vi "Verify File.vi"(5 "Options":T1, 7 "Test VI (caller)":string, 8 "error in":errorcluster, 9 "Extension":string, 10 "Path to Binary File to Verify":path) -> (0 "error out":errorcluster, 1 "Failure Message":string, 2 "Passed?":bool)   [LabVIEW 2020, in "Approval Tests.lvlib"]
doc: "Performs an approval test.\n\nThe first call, the test passes and the test data is written to the approved file.\n\nOn subsequent runs the test data is compared to the contents of the approved file.\nIf it is a match, the test passes.\nIf it is not a match, the test fails and the test data is written to the actual file.\n\nAt the point the user can diff the approved and actual files and determine if they approve of the changes or not. If they approve, they replace the old approved file with the actual file. \n\nNOTE: You should keep the approved files in Source Code Control. You should ignore *.actual in your .gitignore file - there is no need to store those."
uses:
  Approval Tests.lvlib
  Options.ctl
  Reporter/Reporter.lvclass
  Printer/Printer.lvclass
  <vilib>/SourceControl/sccapi/SCCAPI VI Compare Options.ctl
  <vilib>/security/Message Digest/API/Instances/File/SHA-256 File Checksum.vi
  <vilib>/SourceControl/sccapi/NI_SCC.lvlib
  <vilib>/security/Message Digest/API/NI_Message Digest API.lvlib
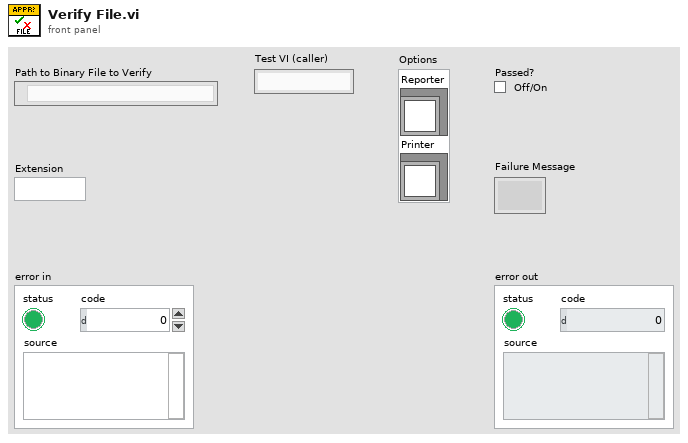
[diagram p1: front panel]
types:
  T1 = typedef "Approval Tests.lvlib/Options.ctl" = cluster{"Reporter":refnum<class "Reporter.lvclass">, "Printer":refnum<class "Printer.lvclass">}
  T2 = typedef "NI_SCC.lvlib/SCCAPI VI Compare Options.ctl" = cluster{"VI Attributes":bool, "Front Panel":bool, "FP position/size":bool, "Block Diagram":bool, "BD cosmetic":bool, "BD position/size":bool}
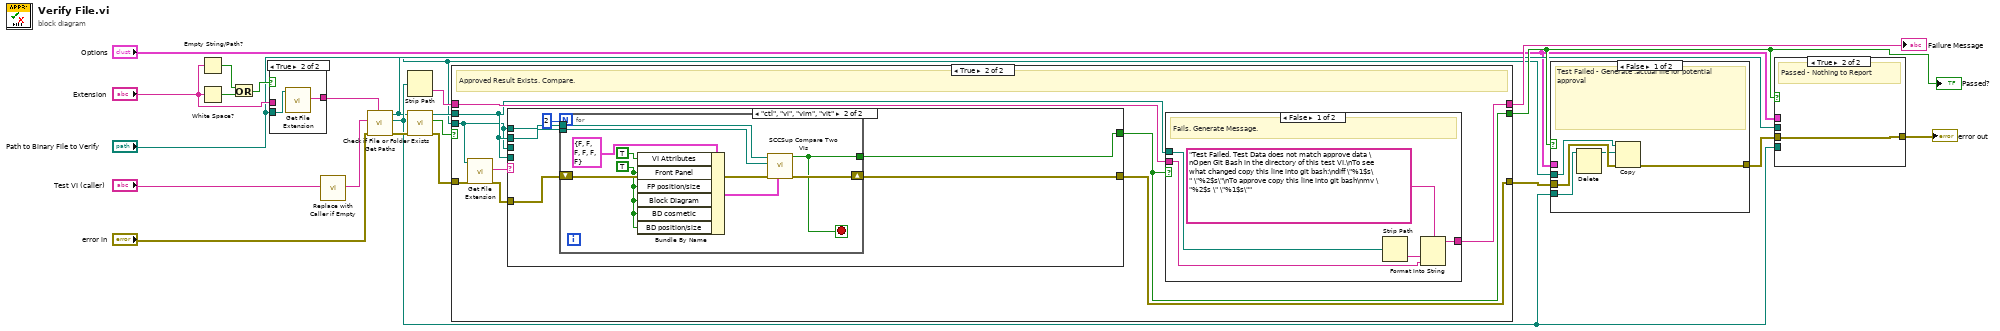
[diagram p0: block diagram]
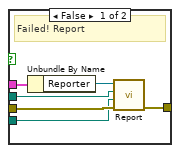
[diagram p3: hidden frame]
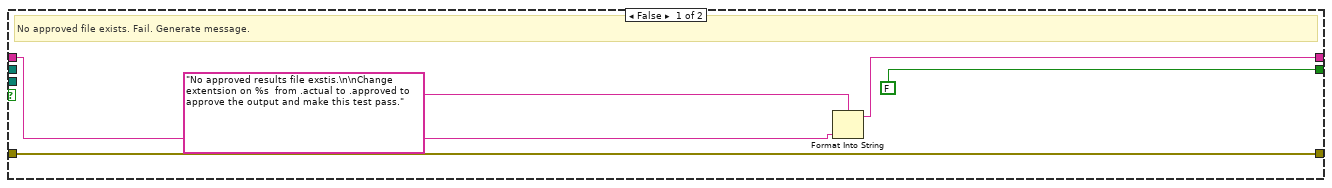
[diagram p5: hidden frame]
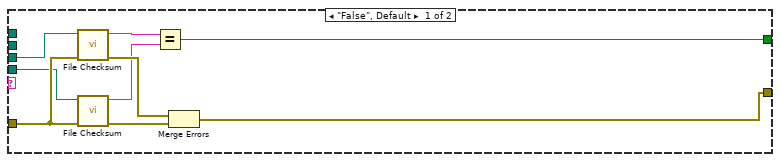
[diagram p6: hidden frame]
diagram:
  n1 = Empty String/Path?(string/path="Extension") -> (empty?=w6:bool)
  n2 = White Space?(1:"Extension") -> (0:w5:bool)
  n3 = Or(x=w6, y=w5) -> (x .or. y?=w4:bool)
  n4 = case shown="True" w4 {
    tunnel: "Path to Binary File to Verify" -> [_ w25]
    tunnel: [w23 w24] -> w3
    tunnel: "Extension" -> [w23 _]
    frame False {
    }
    frame True {
      n5 = call <vilib>:"Get File Extension.vi"("file"=w25) -> ("lowercase file extension"=w24:string)  [unwired: 6 in, 4 out]
    }
  }
  n6 = call "Replace with Caller if Empty.vi"("Test VI (caller) in"="Test VI (caller)") -> ("Test VI (caller) out"=w7:string)  [unwired: 10 in]
  n7 = call "Get Paths.vi"("Extension(txt)"=w3, "error in"="error in", "VI name"=w7) -> ("error out"=w22:errorcluster, "recived path"=w11:path, "approved path"=w10:path)  [unwired: 6 in]
  n8 = Strip Path(path=w11) -> (name=w13:string)  [unwired: 1 out]
  n9 = call <vilib>:"Check if File or Folder Exists.vi"("error in (no error)"=w22, "path"=w10) -> ("error out"=w21:errorcluster, "file or folder exists?"=w15:bool, "dup path"=w16:path)  [unwired: 7 in]
  n10 = case shown="True" w15 {
    tunnel: [w30 w38] -> w20
    tunnel: w21 -> [w30 w39]
    tunnel: w16 -> [_ w32]
    tunnel: [FALSE ("Passed?") w36] -> w12
    tunnel: [w26 w35] -> w14
    tunnel: w13 -> [w28 w34]
    tunnel: "Path to Binary File to Verify" -> [_ w31]
    frame False {
      # "No approved file exists. Fail. Generate message."
      n11 = Format Into String(format string="No approved results file exstis.\n\nChange extentsion on %s  from .actual to .approved to approve the output and make this test pass.", w28) -> (resulting string=w26:string)  [unwired: 2 in, 1 out]
    }
    frame True {
      # "Approved Result Exists. Compare."
      n12 = call <vilib>:"Get File Extension.vi"("error in (no error)"=w39, "file"=w31) -> ("error out"=w37:errorcluster, "lowercase file extension"=w33:string)  [unwired: 5 in, 3 out]
      n13 = case shown="\"ctl\", \"vi\", \"vim\", \"vit\"" w33 {
        tunnel: [w45 w54] -> w38
        tunnel: [w40 w50] -> w36
        tunnel: w32 -> [_ w52]
        tunnel: w31 -> [_ w51]
        tunnel: w37 -> [w48 w53]
        tunnel: w31 -> [w44 _]
        tunnel: w32 -> [w43 _]
        frame "False", Default {
          n14 = call-poly <vilib>:"File Checksum.vi"("error in"=w48, "path"=w44) -> ("error out"=w46:errorcluster, "digest"=w42:string)  [unwired: 8 in]
          n15 = call-poly <vilib>:"File Checksum.vi"("error in"=w48, "path"=w43) -> ("error out"=w47:errorcluster, "digest"=w41:string)  [unwired: 8 in]
          n16 = Equal?(x=w42, y=w41) -> (x = y?=w40:bool)
          n17 = Merge Errors(w46, w47) -> (w45:errorcluster)
        }
        frame "ctl", "vi", "vim", "vit" {
          n18 = for {
            N: 2 -> [_]
            tunnel: w52 -> [w61]
            tunnel: w51 -> [w60]
            tunnel: [w55] -> w50
            shift-right: [w63] -> w54
            shift-left: w53 -> [w62]
            stop <- w55 stop-if-true
            w57 = TRUE
            n19 = Bundle By Name(cluster=T2 {"VI Attributes"=FALSE, "Front Panel"=FALSE, "FP position/size"=FALSE, "Block Diagram"=FALSE, "BD cosmetic"=FALSE, "BD position/size"=FALSE} ("compare options"), "VI Attributes"=TRUE, "Front Panel"=w57, "FP position/size"=w57, "Block Diagram"=w57, "BD cosmetic"=w57, "BD position/size"=w57) -> (w58:T2)
            n20 = call <vilib>:"SCCSup Compare Two VIs.vi"("compare options"=w58, "error in (no error)"=w62, "Second VI"=w61, "First VI"=w60) -> ("error out"=w63:errorcluster, "Same?"=w55:bool)  [unwired: 5 in, 1 out]
          }
        }
      }
      n21 = case shown="False" w36 {
        tunnel: [w68 _] -> w35
        tunnel: w32 -> [w65 _]
        tunnel: w34 -> [w64 _]
        frame False {
          # "Fails. Generate Message."
          n22 = Strip Path(path=w65) -> (name=w66:string)  [unwired: 1 out]
          n23 = Format Into String(format string="Test Failed. Test Data does not match approve data \nOpen Git Bash in the directory of this test VI.\nTo see what changed copy this line into git bash:\ndiff \"%1$s\" \"%2$s\"\nTo approve copy this line into git bash\nmv \"%2$s \" \"%1$s\"", w66, w64) -> (resulting string=w68:string)  [unwired: 2 in, 1 out]
        }
        frame True {
          # "Passes. No Message Needed.."
        }
      }
    }
  }
  "Passed?" <- w12
  "Failure Message" <- w14
  n24 = case shown="False" w12 {
    tunnel: w20 -> [w73 w74]
    tunnel: [w72 w74] -> w19
    tunnel: w11 -> [w71 _]
    tunnel: "Path to Binary File to Verify" -> [w69 _]
    tunnel: "Options" -> [_ _]
    frame False {
      # "Test Failed - Generate .actual file for potential approval"
      n25 = Delete(path (use dialog)=w71) -> (deleted path=w70:path)  [unwired: 4 in, 2 out]
      n26 = Copy(8:w73, 10:w70, 11:w69) -> (0:w72:errorcluster)  [unwired: 2 in, 2 out]
    }
    frame True {
      # "Passed - no need for .actual file"
    }
  }
  n27 = case shown="True" w12 {
    tunnel: w11 -> [w77 _]
    tunnel: w10 -> [w78 _]
    tunnel: w19 -> [w80 w81]
    tunnel: [w79 w81] -> w18
    tunnel: "Options" -> [w76 _]
    frame False {
      # "Failed! Report"
      n28 = Unbundle By Name(w76) -> ("Reporter"=w75:refnum<class "Reporter.lvclass">)
      n29 = call-dynamic "Report.vi"("error in"=w80, "Received"=w77, "Approved"=w78, "Reporter in"=w75) -> ("error out"=w79:errorcluster)  [unwired: 5 in, 2 out]
    }
    frame True {
      # "Passed - Nothing to Report"
    }
  }
  "error out" <- w18
